vi "Get 1D Time Stamp.vi"(7 "key description":string, 8 "sections":string[](array[string]), 9 "time stamp":timestamp[](array[timestamp]), 11 "info data":string) -> (0 "sections out":string[](array[string]), 1 "key found?":bool, 2 "value":timestamp[](array[timestamp]), 3 "info data out":string)   [LabVIEW 2020, in "infolib.lvlib"]
doc: "Reads horizontal or vertical vector of time stamps. If section is entered it searches the key in the section(s)."
uses:
  infolib.lvlib
  Get 2D Time Stamp.vi
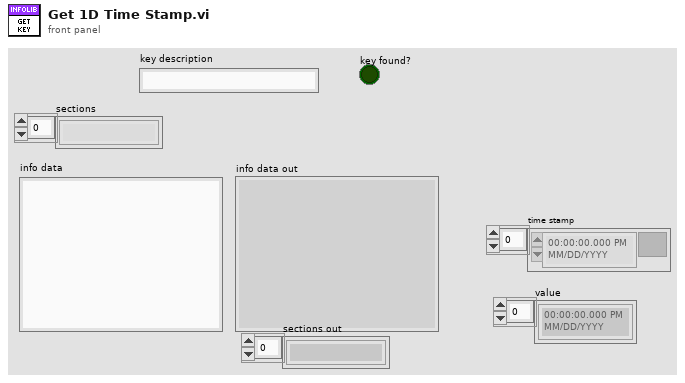
[diagram p1: front panel]
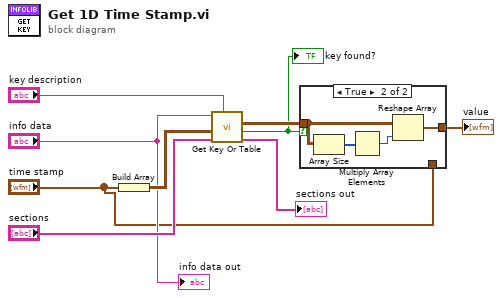
[diagram p0: block diagram]
diagram:
  n1 = Build Array("time stamp") -> (w9:timestamp[][])
  n2 = call-poly "Get Key Or Table.vi"("key description"="key description", "sections"="sections", "time stamp"=w9, "info data"="info data") -> ("sections out"=→"sections out":string[], "key found?"=w1:bool, "value"=w4:timestamp[][])  [unwired: 4 in, 1 out]
  "key found?" <- w1
  n3 = case shown="True" w1 {
    tunnel: w4 -> [_ w12]
    tunnel: [w10 w11] -> w3
    tunnel: "time stamp" -> [w10 _]
    frame False {
    }
    frame True {
      n4 = Array Size(array=w12) -> (size(s)=w13:i32[])
      n5 = Multiply Array Elements(1:w13) -> (0:w14:i32)
      n6 = Reshape Array(w12, w14) -> (w11:timestamp[])
    }
  }
  "value" <- w3
  "info data out" <- "info data"
